vi "p1.vi"() -> ()   [LabVIEW 2021, in "d16.lvlib"]
uses:
  d16.lvlib
  Volcano/Volcano.lvclass
  Volcano/Volcano.lvclass/Volcano.ctl
  AOC/AOC.lvlib
panel:
  in  "Force":bool=TRUE
  in  "Valve":string[](array[string])=["DD", "BB", "JJ", "HH", "EE", "CC"]
  out "Waveform Chart":i32(graph)
  out "iterations":i32=11361
  out "# elements in queue":i32
  in  "Max Time":i32=30
  in  "Example":string="Valve AA has flow rate=0; tunnels lead to valves DD, II, BB\nValve BB has flow rate=13; tunnels lead to valves CC, AA\nValve CC has flow rate=2; tunnels lead to valves DD, BB\nValve DD has flow rate=20; tunnels lead to valves CC, AA, EE\nValve EE has flow rate=3; tunnels lead to valves FF, DD\nValve FF has flow rate=0; tunnels lead to valves EE, GG\nValve GG has flow rate=0; tunnels lead to valves FF, HH\nValve HH has flow rate=22; tunnel leads to valve GG\nValve II has flow rate=0; tunnels lead to valves AA, JJ\nValve JJ has flow rate=21; tunnel leads to valve II"
  in  "Example":bool=TRUE
  out "Answer":u64=1552
  # "2045 is too low"
  # "2183 is with 31"
  # "2067"
  # "3000 is too high"
  # "2051"
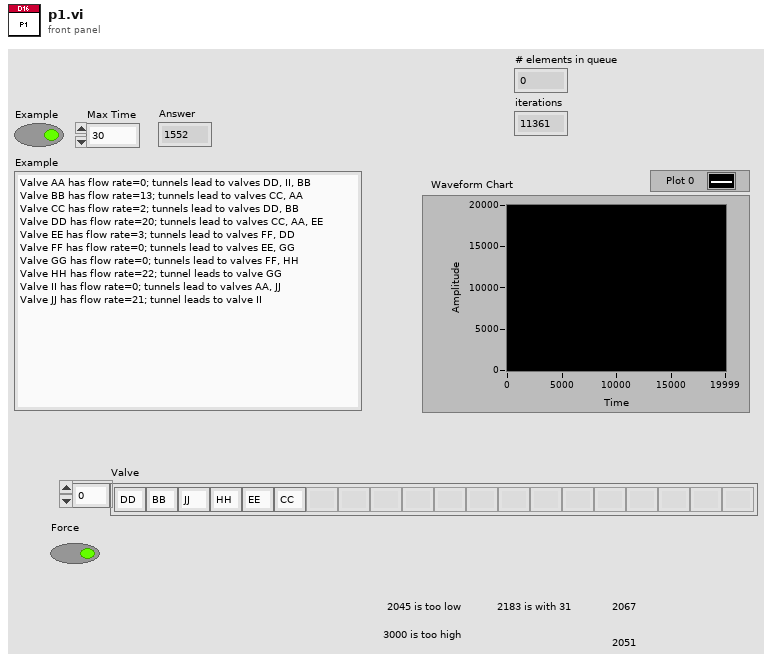
[diagram p1: front panel]
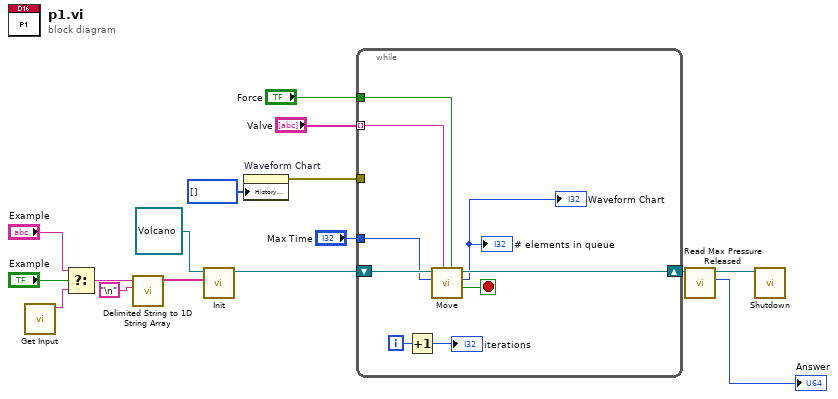
[diagram p0: block diagram]
diagram:
  n1 = call "Get Input.vi"() -> ("Input"=w16:string)  [unwired: 11 in]
  n2 = Select(t="Example", s="Example", f=w16) -> (s? t:f=w15:string)
  n3 = call <vilib>:"Delimited String to 1D String Array.vi"("delimiter"="\n", "delimited string"=w15) -> ("string array"=w10:string[])  [unwired: 9 in]
  n4 = call "Init.vi"("input"=w10, "Volcano in"=refnum<class "Volcano.lvclass"> refnum ("d16.lvlib:Volcano.lvclass")) -> ("Volcano out"=w9:refnum<class "Volcano.lvclass">)  [unwired: 9 in]
  n5 = property on="Waveform Chart" class="WFChart (strict)"("History Data"=i32[] []) -> (error out=w3:errorcluster)  [unwired: 2 in, 1 out]
  n6 = while {
    shift-right: [w24] -> w6
    shift-left: w9 -> [w25]
    tunnel: "Max Time" -> [w23]
    tunnel: w3 -> [_]
    tunnel: "Valve" -> [w18] mode=indexing
    tunnel: "Force" -> [w17]
    i -> [w21]
    stop <- w22 stop-if-true
    n7 = Increment(x=w21) -> (x+1=→"iterations":i32)
    n8 = call "Move.vi"("Force"=w17, "Valve"=w18, "max time"=w23, "Volcano in"=w25) -> ("Finished?"=w22:bool, "# elements in queue"=→"# elements in queue" →"Waveform Chart":i32, "Volcano out"=w24:refnum<class "Volcano.lvclass">)  [unwired: 5 in]
  }
  n9 = call "Read Max Pressure Released.vi"("Volcano in"=w6) -> ("Max Pressure Released"=→"Answer":u64, "Volcano out"=w7:refnum<class "Volcano.lvclass">)  [unwired: 9 in]
  n10 = call "Shutdown.vi"("Volcano in"=w7) -> ()  [unwired: 10 in, 1 out]
